vi "write TBM configuration.vi"(8 "error in":errorcluster, 10 "configuration":refnum<class "TBM configuration.lvclass">, 11 "Systems in":refnum<class "Systems.lvclass">) -> (0 "error out":errorcluster, 3 "Systems out":refnum<class "Systems.lvclass">)   [LabVIEW 2013, in "PL Framework Configuration Tool.lvlib" / "Systems.lvclass"]
uses:
  Systems.lvclass
  <vilib>/NI/Tag Bus Module Framework/root configuration/TBM configuration.lvclass
  Framework Configuration Classes/system configuration/PL_System Configuration.lvclass
  Systems.lvclass/Systems.ctl
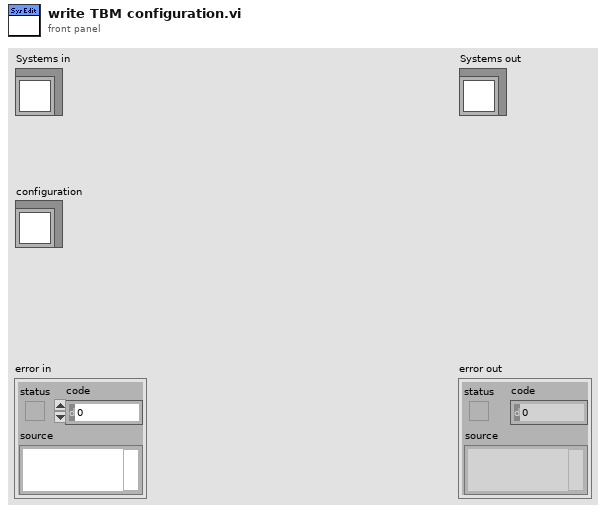
[diagram p1: front panel]
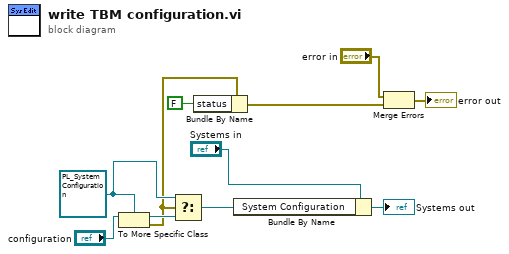
[diagram p0: block diagram]
diagram:
  w8 = refnum<class "PL_System Configuration.lvclass"> refnum ("System Configuration")
  n1 = To More Specific Class(target class=w8, reference="configuration") -> (specific class reference=w7:refnum<class "PL_System Configuration.lvclass">, error out=w3:errorcluster)  [unwired: 1 in]
  n2 = Select(t=w8, s=w3, f=w7) -> (s? t:f=w5:refnum<class "PL_System Configuration.lvclass">)
  n3 = Bundle By Name(cluster=w3, "status"=FALSE) -> (w1:errorcluster)
  n4 = Bundle By Name(cluster="Systems in", "System Configuration"=w5) -> (→"Systems out":refnum<class "Systems.lvclass">)
  n5 = Merge Errors("error in", w1) -> (→"error out":errorcluster)
